vi "Json Tester.vi"() -> ()   [LabVIEW 2021]
uses:
  json class.lvclass
panel:
  out "String":string
  out "DBL 2":dbl
  out "Path":path
  out "DBL":dbl
  out "I32":i32
  out "U32":u32
  out "DBL Array":dbl[](array[numeric])
  out "String Array":string[](array[string])
  out "Item Names 2":string[](array[string])
  out "Item Names":string[](array[string])
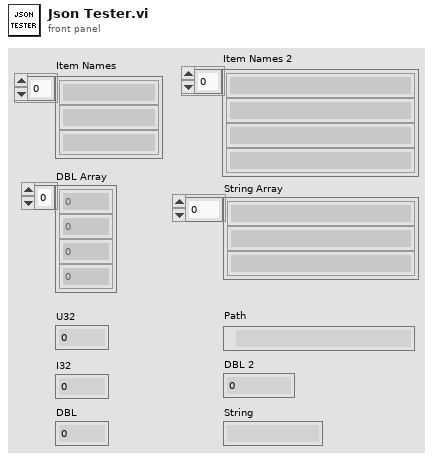
[diagram p1: front panel]
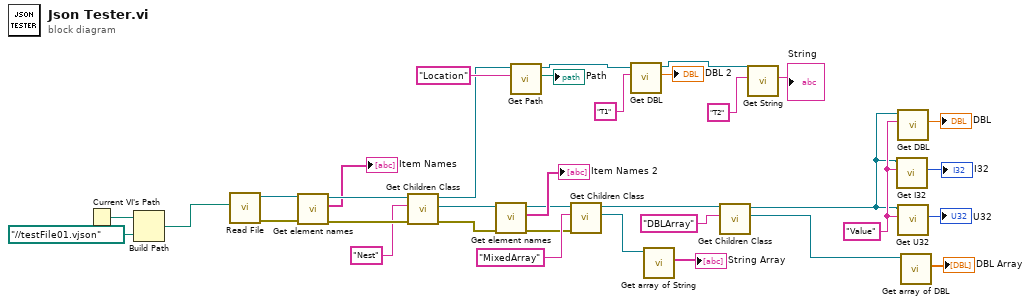
[diagram p0: block diagram]
diagram:
  w12 = "Value" ("Element")
  n1 = Current VI's Path() -> (path=w33:path)
  n2 = Build Path(base path=w33, name or relative path=path "../../testFile01.vjson") -> (appended path=w31:path)
  n3 = call "Read File.vi"("Path"=w31) -> ("error out"=w34:errorcluster, "json class out"=w35:refnum<class "json class.lvclass">)  [unwired: 9 in]
  n4 = call-dynamic "Get element names.vi"("error in (no error)"=w34, "json class in"=w35) -> ("error out"=w29:errorcluster, "Item Names"=→"Item Names":string[], "json class out"=w30:refnum<class "json class.lvclass">)  [unwired: 7 in]
  n5 = call-dynamic "Get Children Class.vi"("error in (no error)"=w29, "Element"="Nest", "json class in"=w30) -> ("error out"=w25:errorcluster, "Children class"=w26:refnum<class "json class.lvclass">, "json class out"=w7:refnum<class "json class.lvclass">)  [unwired: 6 in]
  n6 = call-dynamic "Get element names.vi"("error in (no error)"=w25, "json class in"=w26) -> ("error out"=w20:errorcluster, "Item Names"=→"Item Names 2":string[], "json class out"=w22:refnum<class "json class.lvclass">)  [unwired: 7 in]
  n7 = call "Get Path.vi"("Name"="Location", "json class in"=w7) -> ("Path"=→"Path":path, "json class out"=w6:refnum<class "json class.lvclass">)  [unwired: 7 in, 1 out]
  n8 = call-dynamic "Get Children Class.vi"("error in (no error)"=w20, "Element"="MixedArray", "json class in"=w22) -> ("Children class"=w19:refnum<class "json class.lvclass">, "json class out"=w18:refnum<class "json class.lvclass">)  [unwired: 6 in, 1 out]
  n9 = call "Get DBL.vi"("Name"="T1", "json class in"=w6) -> ("DBL"=→"DBL 2":dbl, "json class out"=w3:refnum<class "json class.lvclass">)  [unwired: 7 in, 1 out]
  n10 = call "Get array of String.vi"("json class in"=w19) -> ("String Array"=→"String Array":string[])  [unwired: 8 in, 2 out]
  n11 = call-dynamic "Get Children Class.vi"("Element"="DBLArray", "json class in"=w18) -> ("Children class"=w16:refnum<class "json class.lvclass">, "json class out"=w10:refnum<class "json class.lvclass">)  [unwired: 7 in, 1 out]
  n12 = call "Get String.vi"("Name"="T2", "json class in"=w3) -> ("String"=→"String":string)  [unwired: 7 in, 2 out]
  n13 = call "Get I32.vi"("Name"=w12, "json class in"=w10) -> ("I32"=→"I32":i32)  [unwired: 7 in, 2 out]
  n14 = call "Get DBL.vi"("Name"=w12, "json class in"=w10) -> ("DBL"=→"DBL":dbl)  [unwired: 7 in, 2 out]
  n15 = call "Get U32.vi"("Name"=w12, "json class in"=w10) -> ("U32"=→"U32":u32)  [unwired: 7 in, 2 out]
  n16 = call "Get array of DBL.vi"("json class in"=w16) -> ("DBL Array"=→"DBL Array":dbl[])  [unwired: 8 in, 2 out]
